vi "get_ip.vi"(8 "error in (no error)":errorcluster, 9 "string in":string) -> (0 "error out":errorcluster, 1 "edited string out":string, 2 "ip address out":string)   [LabVIEW 2010, in "ErrorController.lvclass"]
uses:
  ErrorController.lvclass
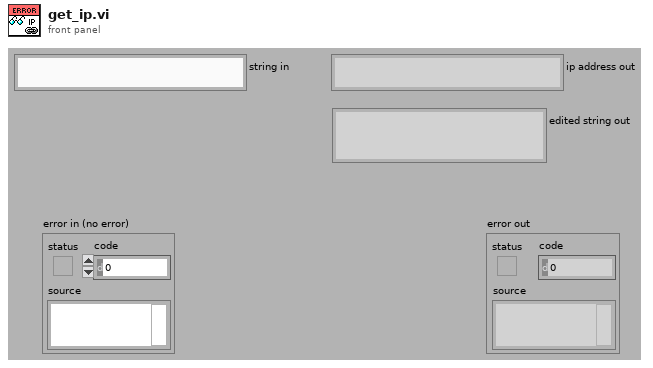
[diagram p1: front panel]
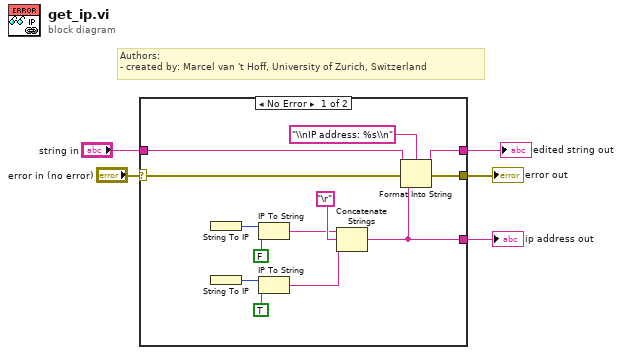
[diagram p0: block diagram]
diagram:
  # "Authors: \n- created by: Marcel van 't Hoff, University of Zurich, Switzerland"
  n1 = case shown="No Error" "error in (no error)" {
    selector: "error in (no error)" -> [w11 w20]
    tunnel: [w10 w20] -> w4
    tunnel: [w7 _] -> w3
    tunnel: "string in" -> [w9 w19]
    tunnel: [w8 w19] -> w1
    frame No Error {
      n2 = String To IP() -> (0:w12:u32)  [unwired: 1 in]
      n3 = String To IP() -> (0:w17:u32)  [unwired: 1 in]
      n4 = IP To String(1:FALSE ("dot notation? (F)"), 2:w12) -> (0:w14:string)
      n5 = IP To String(1:TRUE ("dot notation? (F)"), 2:w17) -> (0:w18:string)
      n6 = Concatenate Strings(w14, "\r", w18) -> (w7:string)
      n7 = Format Into String(format string="\\nIP address: %s\\n", initial string=w9, error in=w11, w7) -> (resulting string=w8:string, error out=w10:errorcluster)
    }
    frame Error {
    }
  }
  "error out" <- w4
  "ip address out" <- w3
  "edited string out" <- w1
